vi "LCP Stop All Pumps.vi"(8 "error in (no error)":errorcluster caption="Fehler (Eingang, kein Fehler)") -> (0 "error out":errorcluster caption="Fehler (Ausgang)")   [LabVIEW 2021, in "labbCAN_Pump_API.lvlib"]
doc: "LCP_Func long LCP_CALL LCP_StopAllPumps();"
uses:
  labbCAN_Pump_API.lvlib
  labbCAN_Pump_API.dll
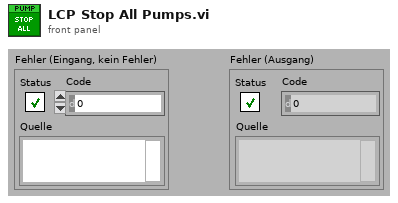
[diagram p1: front panel]
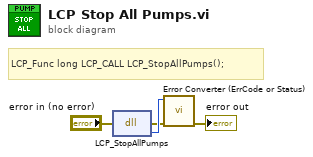
[diagram p0: block diagram]
diagram:
  # "LCP_Func long LCP_CALL LCP_StopAllPumps();"
  n1 = dll-call lib="C:/Users/olaja/AppData/Local/CETONI_SDK/labbCAN_Pump_API.*" fn="LCP_StopAllPumps"(error in="error in (no error)") -> (error out=w2:errorcluster, w3:i32)  [unwired: 2 in, 1 out]
  n2 = call "Error Converter (ErrCode or Status).vi"("error in (no error)"=w2, "error code"=w3) -> ("error out"=→"error out":errorcluster)  [unwired: 9 in]
